vi "UTC_to_Timestamp.vi"(11 "UTC Time":u64) -> (2 "Timestamp (s)":dbl format="%#_8g", 3 "Timestamp":timestamp format="%<%.6X\n%x>T")   [LabVIEW 2020]
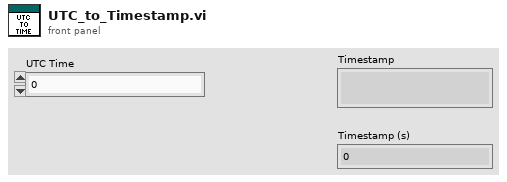
[diagram p1: front panel]
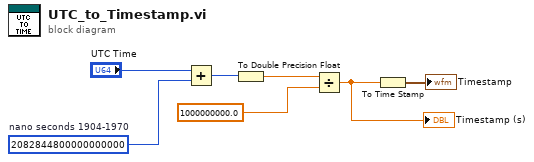
[diagram p0: block diagram]
diagram:
  w6 = u64 2082844800000000000  # nano seconds 1904-1970
  n1 = Add(x="UTC Time", y=w6) -> (x+y=w3:u64)
  n2 = To Double Precision Float(number=w3) -> (double precision float=w5:dbl)
  n3 = Divide(x=w5, y=1000000000.0) -> (x/y=w2:dbl)
  "Timestamp (s)" <- w2
  n4 = To Time Stamp(1:w2) -> (0:→"Timestamp":timestamp)
